vi "pixel counter z.vi"(6 "stim delay":u16=5, 7 "stim duration":u16=20, 8 "counter cluster in":T2, 9 "scanning":bool, 10 "scan specification":T3, 11 "tag lens trigger":bool) -> (0 "counter cluster out":T2, 1 "trigger diagnostics":T1, 2 "fly back":bool, 3 "acquire":bool, 4 "new line":bool, 5 "stim light window":bool)   [LabVIEW 2010]
uses:
  scan_specification_tagResonant.ctl
  counter_cluster_tagResonant.ctl
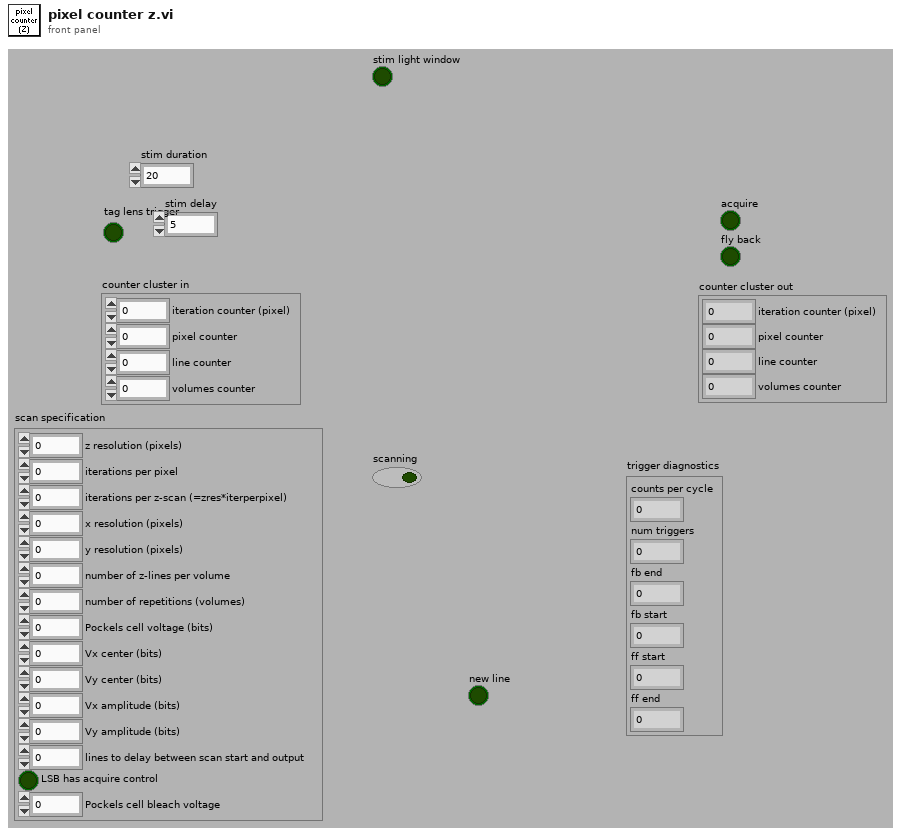
[diagram p1: front panel]
types:
  T1 = cluster{"counts per cycle":u16, "num triggers":u32, "fb end":u16, "fb start":u16, "ff start":u16, "ff end":u16}
  T2 = typedef "counter_cluster_tagResonant.ctl" = cluster{"iteration counter (pixel)":u16, "pixel counter":u16, "line counter":i16, "volumes counter":u16}
  T3 = typedef "scan_specification_tagResonant.ctl" = cluster{"z resolution (pixels)":u16, "iterations per pixel":u16, "iterations per z-scan (=zres*iterperpixel)":u16, "x resolution (pixels)":u16, "y resolution (pixels)":u16, "number of z-lines per volume":u16, "number of repetitions (volumes)":i32, "Pockels cell voltage (bits)":i16, "Vx center (bits)":i16, "Vy center (bits)":i16, "Vx amplitude (bits)":i16, "Vy amplitude (bits)":i16, "lines to delay between scan start and output":u16, "LSB has acquire control":bool, "Pockels cell bleach voltage":i16}
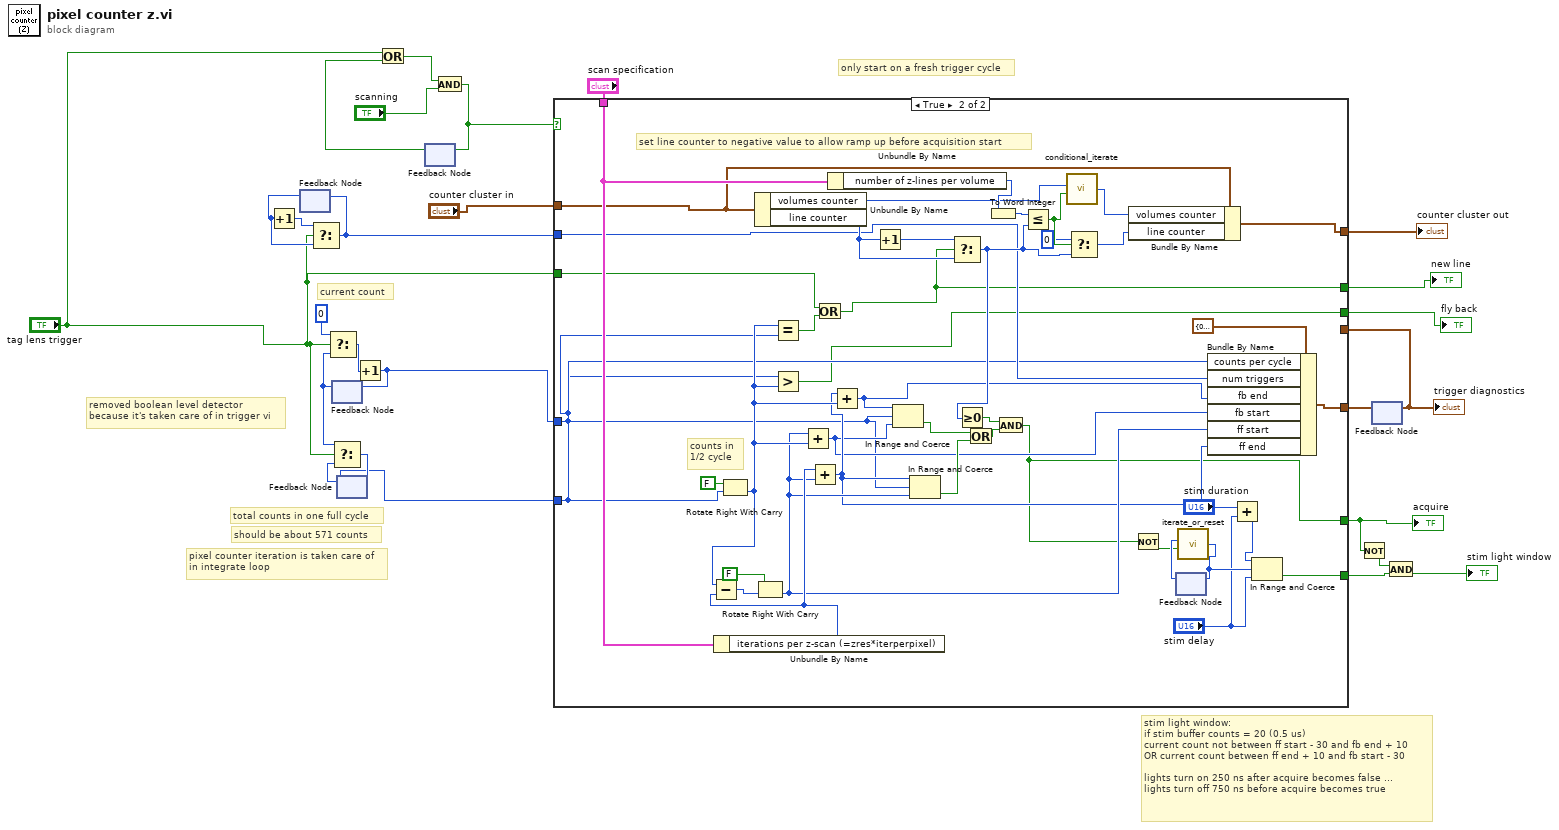
[diagram p0: block diagram]
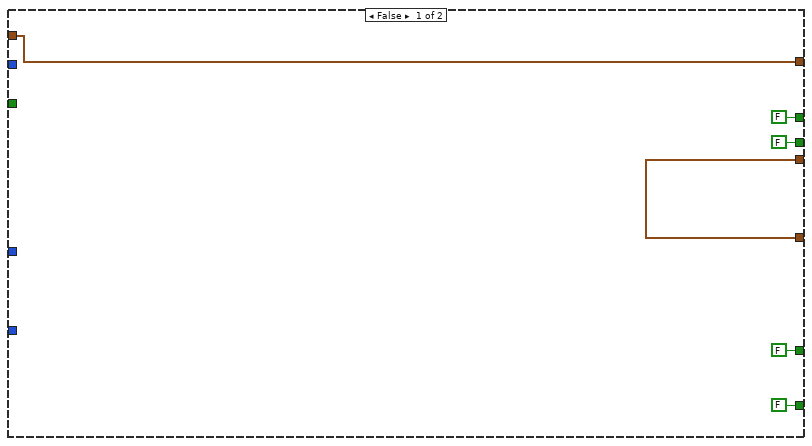
[diagram p2: hidden frame]
diagram:
  # "should be about 571 counts"
  # "stim light window:\nif stim buffer counts = 20 (0.5 us)\ncurrent count not between ff start - 30 and fb end + 10\nOR current count between ff end + 10 and fb start - 30\n\nlights turn on 250 ns after acquire becomes false ...\nlights turn off 750 ns before acquire becomes true"
  # "pixel counter iteration is taken care of\nin integrate loop"
  # "removed boolean level detector\nbecause it's taken care of in trigger vi"
  # "only start on a fresh trigger cycle"
  # "total counts in one full cycle"
  # "current count"
  n1 = feedback #1() -> (w17:u32)  [unwired: 1 in]
  n2 = Increment(x=w17) -> (x+1=w18:u32)
  n3 = Select(t=w18, s="tag lens trigger", f=w17) -> (s? t:f=w16:u32)
  n4 = feedback-in #1(w16) -> ()
  n5 = feedback #2() -> (w23:u16)  [unwired: 1 in]
  n6 = Select(t=u16 0, s="tag lens trigger", f=w23) -> (s? t:f=w24:u16)
  n7 = feedback #3() -> (w15:u16)  [unwired: 1 in]
  n8 = Select(t=w23, s="tag lens trigger", f=w15) -> (s? t:f=w22:u16)
  n9 = feedback-in #3(w22) -> ()
  n10 = Increment(x=w24) -> (x+1=w21:u16)
  n11 = feedback-in #2(w21) -> ()
  n12 = feedback #4() -> (w12:bool)  [unwired: 1 in]
  n13 = Or(x="tag lens trigger", y=w12) -> (x .or. y?=w13:bool)
  n14 = And(x=w13, y="scanning") -> (x .and. y?=w11:bool)
  n15 = feedback-in #4(w11) -> ()
  n16 = feedback #5() -> (w8:T1)  [unwired: 1 in]
  "trigger diagnostics" <- w8
  n17 = case shown="True" w11 {
    tunnel: w21 -> [_ w40]
    tunnel: "scan specification" -> [_ w66]
    tunnel: [w31 w60] -> w19
    tunnel: [FALSE w38] -> w3
    tunnel: "tag lens trigger" -> [_ w52]
    tunnel: w16 -> [_ w50]
    tunnel: w15 -> [_ w49]
    tunnel: [w29 w48] -> w9
    tunnel: "counter cluster in" -> [w31 w47]
    tunnel: w8 -> [w29 _]
    tunnel: [FALSE w46] -> w6
    tunnel: [FALSE w45] -> w5
    tunnel: [FALSE w32] -> w4
    frame False {
    }
    frame True {
      # "set line counter to negative value to allow ramp up before acquisition start"
      # "counts in \n1/2 cycle"
      n18 = Unbundle By Name(w66) -> ("iterations per z-scan (=zres*iterperpixel)"=w69:u16)
      n19 = Rotate Right With Carry(2:w49, 3:FALSE ("carry")) -> (0:w68:u16)  [unwired: 1 out]
      n20 = Subtract(x=w68, y=w69) -> (x-y=w73:u16)
      n21 = Unbundle By Name(w47) -> ("volumes counter"=w63:u16, "line counter"=w59:i16)
      n22 = Rotate Right With Carry(2:w73, 3:FALSE ("carry")) -> (0:w44:u16)  [unwired: 1 out]
      n23 = Equal?(x=w68, y=w40) -> (x = y?=w67:bool)
      n24 = Greater?(x=w40, y=w68) -> (0:w45:bool)
      n25 = Add(x=w44, y=w68) -> (x+y=w41:u16)
      n26 = Add(x=w69, y=w44) -> (x+y=w42:u16)
      n27 = Or(x=w52, y=w67) -> (x .or. y?=w46:bool)
      n28 = Unbundle By Name(w66) -> ("number of z-lines per volume"=w65:u16)
      n29 = Add(x=w42, y=w68) -> (x+y=w43:u16)
      n30 = Increment(x=w59) -> (x+1=w58:i16)
      n31 = In Range and Coerce(upper limit=w43, x=w40, lower limit=w41) -> (In Range?=w71:bool)  [unwired: 1 out]
      n32 = In Range and Coerce(upper limit=w42, x=w40, lower limit=w44) -> (In Range?=w70:bool)  [unwired: 1 out]
      n33 = Select(t=w58, s=w46, f=w59) -> (s? t:f=w55:i16)
      n34 = Greater Or Equal To 0?(x=w55) -> (x >= 0?=w54:bool)
      n35 = Or(x=w71, y=w70) -> (x .or. y?=w53:bool)
      n36 = To Word Integer(number=w65) -> (16bit integer=w56:i16)
      n37 = And(x=w54, y=w53) -> (x .and. y?=w38:bool)
      n38 = Less Or Equal?(x=w56, y=w55) -> (x <= y?=w64:bool)
      n39 = call "conditional_iterate.vi"("iterate?"=w64, "number in"=w63) -> ("number out"=w62:u16)  [unwired: 4 in]
      n40 = Select(t=i16 0, s=w64, f=w55) -> (s? t:f=w61:i16)
      n41 = Bundle By Name(cluster=w47, "volumes counter"=w62, "line counter"=w61) -> (w60:T2)
      n42 = Not(x=w38) -> (.not. x?=w33:bool)
      n43 = feedback #6() -> (w39:u16)  [unwired: 1 in]
      n44 = call "iterate_or_reset.vi"("iterate?"=w33, "number in"=w39) -> ("number out"=w37:u16)  [unwired: 4 in]
      n45 = feedback-in #6(w37) -> ()
      n46 = Bundle By Name(cluster=T1 {"counts per cycle"=0, "num triggers"=0, "fb end"=0, "fb start"=0, "ff start"=0, "ff end"=0} ("trigger diagnostics"), "counts per cycle"=w49, "num triggers"=w50, "fb end"=w43, "fb start"=w41, "ff start"=w44, "ff end"=w42) -> (w48:T1)
      n47 = Add(x="stim duration", y="stim delay") -> (x+y=w34:u16)
      n48 = In Range and Coerce(upper limit=w34, x=w37, lower limit="stim delay") -> (In Range?=w32:bool)  [unwired: 1 out]
    }
  }
  "acquire" <- w3
  "counter cluster out" <- w19
  "new line" <- w6
  "fly back" <- w5
  n49 = Not(x=w3) -> (.not. x?=w1:bool)
  n50 = feedback-in #5(w9) -> ()
  n51 = And(x=w1, y=w4) -> (x .and. y?=→"stim light window":bool)
